vi "checkFinishPenaltyEnemyPlayVSS.vi"(8 "error in (no error)":errorcluster, 10 "Game in":refnum<class "Game.lvclass">, 11 "PenaltyEnemyPlayVSS in":refnum<class "PenaltyEnemyPlayVSS.lvclass">) -> (0 "error out":errorcluster, 2 "result":bool, 3 "PenaltyEnemyPlayVSS out":refnum<class "PenaltyEnemyPlayVSS.lvclass">)   [LabVIEW 2023, in "PenaltyEnemyPlayVSS.lvclass"]
uses:
  PenaltyEnemyPlayVSS.lvclass
  Game_class/Game.lvclass
  Game_class/Game.lvclass/Game.ctl
  Events_class/Events.lvclass/Events.ctl
  Game_class/Read Referee.vi
  Game_class/Read EventsRef.vi
  Events_class/Read ball_out.vi
  Events_class/Read touch.vi
  Events_class/Read id_touch.vi
  Events_class/Read ball_out_of_vision.vi
  Referee_class/Referee.lvclass
  Events_class/Events.lvclass
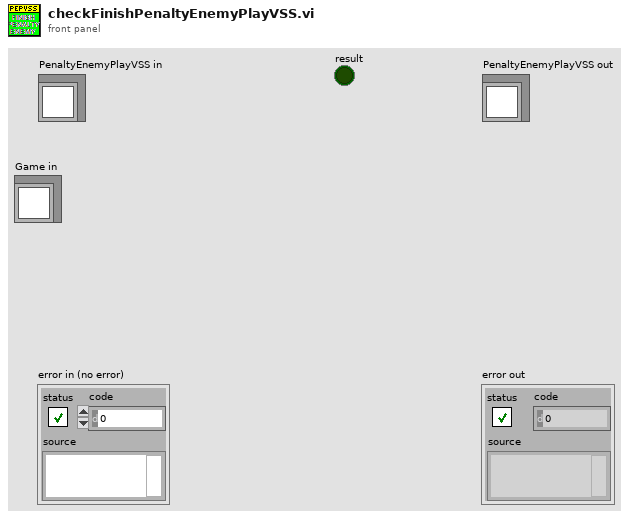
[diagram p1: front panel]
types:
  T1 = enum16{"AUTO", "GAME_ON", "STOP", "KICKOFF", "FREE_BALL", "GOAL_KICK", "PENALTY_KICK", "FREE_KICK"}
  T2 = typedef "Command.ctl" = enum16{"AUTO", "GAME_ON", "STOP", "HALT", "KICKOFF_ALLY", "KICKOFF_ENEMY", "FREE_BALL", "GOAL_KICK_ENEMY", "GOAL_KICK_ALLY", "PENALTY_KICK_ENEMY", "PENALTY_KICK_ALLY", "FREE_KICK"}
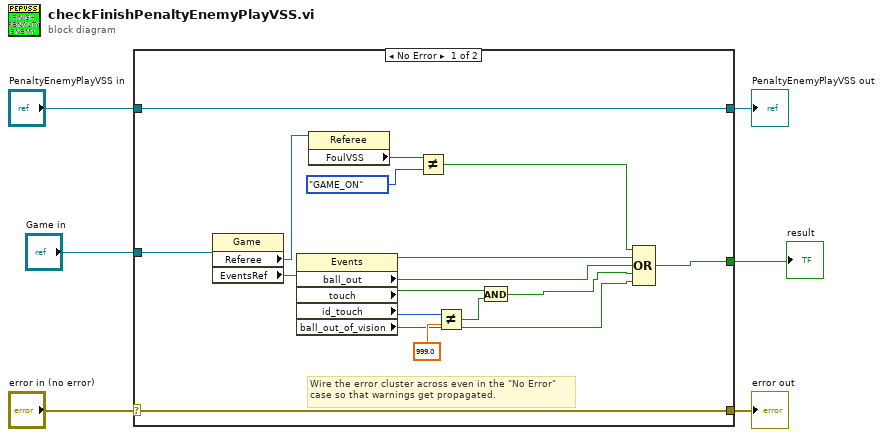
[diagram p0: block diagram]
diagram:
  n1 = case shown="No Error" "error in (no error)" {
    selector: "error in (no error)" -> [w21 w24]
    tunnel: [w21 w24] -> w5
    tunnel: [w22 w23] -> w3
    tunnel: "PenaltyEnemyPlayVSS in" -> [w22 w23]
    tunnel: "Game in" -> [w20 _]
    tunnel: [w18 _] -> w1
    frame No Error {
      # "Wire the error cluster across even in the \"No Error\"\ncase so that warnings get propagated."
      n2 = property class="Game"(reference=w20) -> ("Referee"=w17:refnum<class "Referee.lvclass">, "EventsRef"=w19:refnum<class "Events.lvclass">)  [unwired: 1 in, 2 out]
      n3 = property class="Events"(reference=w19) -> ("ball_out"=w9:bool, "touch"=w11:bool, "id_touch"=w13:i32, "ball_out_of_vision"=w8:bool)  [unwired: 1 in, 2 out]
      n4 = property class="Referee"(reference=w17) -> ("FoulVSS"=w16:T2)  [unwired: 1 in, 2 out]
      n5 = Not Equal?(x=w16, y=T1."GAME_ON") -> (x != y?=w14:bool)
      n6 = Not Equal?(x=w13, y=999.0) -> (x != y?=w10:bool)
      n7 = And(x=w11, y=w10) -> (x .and. y?=w7:bool)
      n8 = Compound Arithmetic op=OR(w14, w9, w9, w7, w8) -> (w18:bool)
    }
    frame Error {
    }
  }
  "error out" <- w5
  "PenaltyEnemyPlayVSS out" <- w3
  "result" <- w1
